vi "ExtractSeqWF.vi"(4 "yee delay":sgl, 5 "Correct Delay?":bool=TRUE, 6 "Acqiris delay":dbl, 7 "String":string, 8 "Offset":i32=11, 9 "Byte Swap":bool=TRUE) -> (1 "vert gain":sgl format="%.2e", 2 "Data Pts":i32, 3 "Data":i8[][](array[numeric]))   [LabVIEW 2022 SP3]
uses:
  -DigitizerRoutines/DigitizerGlobals.vi
panel:
  out "Hor offset":dbl format="%.2e"
  out "Trig Offset":dbl[](array[numeric]) format="%.2e"
  out "Trig Time":dbl[](array[numeric]) format="%.2e"
  out "#Data Bytes":i32
  out "Trig Time Array":i32
  out "Usr Text":i32
  out "Pts Per Screen":i32
  out "Nom Seg Count":i16
  out "WaveDesc":i32
  out "# of Segs":i32
  out "substring":string
  out "Nom bits":i32
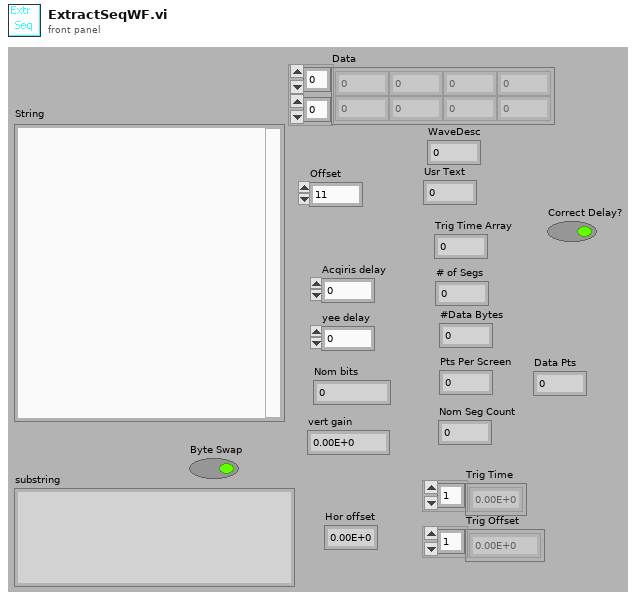
[diagram p1: front panel]
types:
  T1 = typedef "DigitizerSettings.ctl" = cluster{"Digitizer delay (us) ":dbl, "rf points per line":i32, "lines per plane":i32, "Samp Rate (Hz)":dbl, "Additional dig delay (us)":dbl, "Voltage Scale":dbl, "Pre-Looks":i32, "Offset delay (us)":dbl, "bits A/D":i8, "Avg Num":i32, "DigTimeOut":sgl, "Rel Dig Delay":sgl, "Dig Ch":i32, "LeCroyCluster":cluster{"LeCroy Channels":bool[], "LC read pt offset":dbl, "Sweep Avg":bool}, "Main Digitizer":T2, "Dig Config":T3, "Digitizer ID Cluster":T4, "Trigger Settings":cluster{"Trig Source":u16, "Trig Coupling":u16, "Trig Slope":u16, "Level (mV)":dbl}, "Bulk Acq":bool, "Bulk Start Indexes":i32[], "Data Ref RF":refnum<data-value>, "NI ID/Channel":cluster{"NI ID":refnum<k15>, "NI CH":i32}[], "Total Dig CH":i32, "Xtra Ann Trig delay (us)":dbl, "Fix Z Delay?":bool, "One Way Transmission?":bool, "Data Ref Log":refnum<data-value>}
  T2 = typedef "Digitizer.ctl" = enum16{"Acqiris Digitizer", "NI Digitizer", "LeCroy", "GaGe", "AlazarTech", "No Digitizer", "Teledyne"}
  T3 = typedef "DigConfig.ctl" = enum16{"Single channel", "2 Chans w/ 2 Acqiris", "2 Chans w/ 1 Acqiris", "5-CH Pulser New", "5-CH pulser w/ ann array", "5-pass style ann array", "Empty"}
  T4 = typedef "DigitizerID.ctl" = cluster{"Acqiris/Alazar/SP ID":u32[], "NI Instr Handles":refnum<k15>[], "LeCroy VISA":refnum<visa-resource-name>, "GaGe Handle":cluster{"Handle":u32, "Sample size":u32, "Resolution":i32, "Offset":i32, "Channels":u32, "Boards":u32}, "ATS Ref":string, "Acqiris Address":string[], "ADQRef":refnum<k24>, "adq_cu_ptr":refnum<k24>}
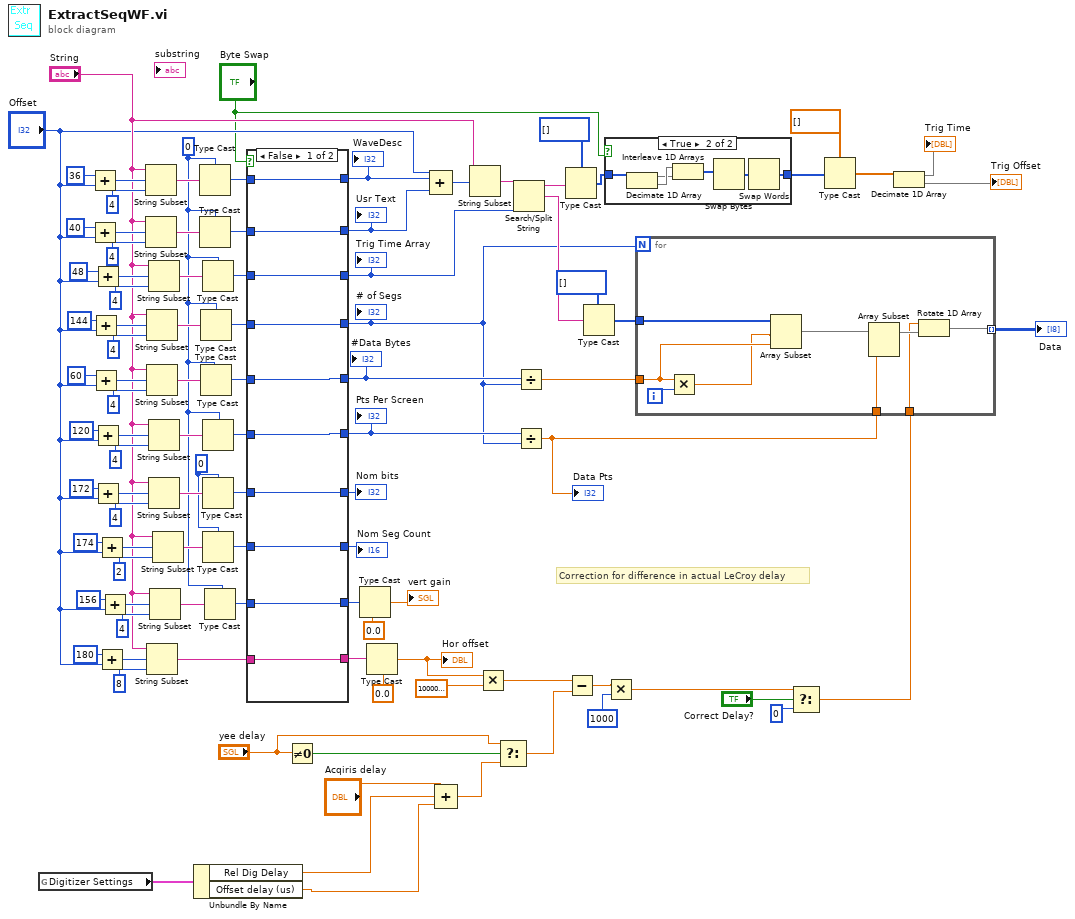
[diagram p0: block diagram]
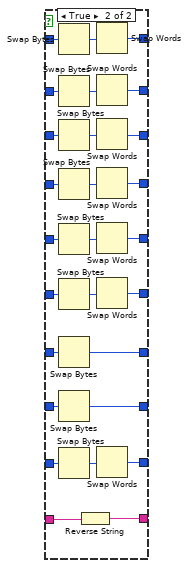
[diagram p3: hidden frame]
diagram:
  w17 = i16 0
  w27 = 0
  # "Correction for difference in actual LeCroy delay"
  n1 = global read "DigitizerGlobals.vi" "Digitizer Settings"() -> (w1:T1)
  n2 = Add(x=36, y="Offset") -> (x+y=w98:i32)
  n3 = Add(x=40, y="Offset") -> (x+y=w93:i32)
  n4 = Add(x=144, y="Offset") -> (x+y=w88:i32)
  n5 = Add(x=60, y="Offset") -> (x+y=w83:i32)
  n6 = Add(x=48, y="Offset") -> (x+y=w59:i32)
  n7 = Add(x=120, y="Offset") -> (x+y=w78:i32)
  n8 = Add(x=172, y="Offset") -> (x+y=w73:i32)
  n9 = Add(x=174, y="Offset") -> (x+y=w68:i32)
  n10 = Add(x=180, y="Offset") -> (x+y=w38:i32)
  n11 = Add(x=156, y="Offset") -> (x+y=w63:i32)
  n12 = String Subset(string="String", offset (0)=w98, length (rest)=4) -> (substring=w96:string)
  n13 = String Subset(string="String", offset (0)=w93, length (rest)=4) -> (substring=w91:string)
  n14 = String Subset(string="String", offset (0)=w88, length (rest)=4) -> (substring=w86:string)
  n15 = String Subset(string="String", offset (0)=w83, length (rest)=4) -> (substring=w81:string)
  n16 = String Subset(string="String", offset (0)=w38, length (rest)=8) -> (substring=w15:string)
  n17 = String Subset(string="String", offset (0)=w59, length (rest)=4) -> (substring=w57:string)
  n18 = String Subset(string="String", offset (0)=w78, length (rest)=4) -> (substring=w76:string)
  n19 = String Subset(string="String", offset (0)=w73, length (rest)=4) -> (substring=w71:string)
  n20 = String Subset(string="String", offset (0)=w63, length (rest)=4) -> (substring=w62:string)
  n21 = String Subset(string="String", offset (0)=w68, length (rest)=2) -> (substring=w66:string)
  n22 = Unbundle By Name(w1) -> ("Rel Dig Delay"=w2:sgl, "Offset delay (us)"=w3:dbl)
  n23 = Type Cast(type=w27, x=w96) -> (*(type *) &x=w97:i32)
  n24 = Type Cast(type=w27, x=w91) -> (*(type *) &x=w92:i32)
  n25 = Type Cast(type=w27, x=w86) -> (*(type *) &x=w87:i32)
  n26 = Type Cast(type=w27, x=w81) -> (*(type *) &x=w82:i32)
  n27 = Type Cast(type=w27, x=w57) -> (*(type *) &x=w58:i32)
  n28 = Type Cast(type=w27, x=w76) -> (*(type *) &x=w77:i32)
  n29 = Type Cast(type=w17, x=w71) -> (*(type *) &x=w72:i16)
  n30 = Type Cast(type=w17, x=w66) -> (*(type *) &x=w67:i16)
  n31 = Type Cast(type=w27, x=w62) -> (*(type *) &x=w44:i32)
  n32 = case shown="False" "Byte Swap" {
    tunnel: w97 -> [w110 w136]
    tunnel: w92 -> [w109 w134]
    tunnel: w87 -> [w107 w132]
    tunnel: w82 -> [w106 w130]
    tunnel: w77 -> [w105 w128]
    tunnel: w72 -> [w104 w127]
    tunnel: w67 -> [w103 w126]
    tunnel: w58 -> [w108 w123]
    tunnel: [w110 w122] -> w55
    tunnel: [w109 w121] -> w54
    tunnel: [w108 w120] -> w51
    tunnel: w44 -> [w102 w119]
    tunnel: [w102 w118] -> w43
    tunnel: [w106 w117] -> w33
    tunnel: [w105 w116] -> w32
    tunnel: [w107 w115] -> w31
    tunnel: [w103 w114] -> w29
    tunnel: [w104 w113] -> w26
    tunnel: w15 -> [w101 w112]
    tunnel: [w101 w111] -> w14
    frame False {
    }
    frame True {
      n33 = Swap Bytes(anything=w136) -> (byte swapped=w137:i32)
      n34 = Swap Bytes(anything=w134) -> (byte swapped=w135:i32)
      n35 = Swap Bytes(anything=w123) -> (byte swapped=w124:i32)
      n36 = Swap Bytes(anything=w132) -> (byte swapped=w133:i32)
      n37 = Swap Bytes(anything=w130) -> (byte swapped=w131:i32)
      n38 = Swap Bytes(anything=w128) -> (byte swapped=w129:i32)
      n39 = Swap Bytes(anything=w127) -> (byte swapped=w113:i16)
      n40 = Swap Bytes(anything=w126) -> (byte swapped=w114:i16)
      n41 = Swap Bytes(anything=w119) -> (byte swapped=w125:i32)
      n42 = Reverse String(1:w112) -> (0:w111:string)
      n43 = Swap Words(1:w137) -> (0:w122:i32)
      n44 = Swap Words(1:w135) -> (0:w121:i32)
      n45 = Swap Words(1:w124) -> (0:w120:i32)
      n46 = Swap Words(1:w133) -> (0:w115:i32)
      n47 = Swap Words(1:w131) -> (0:w117:i32)
      n48 = Swap Words(1:w129) -> (0:w116:i32)
      n49 = Swap Words(1:w125) -> (0:w118:i32)
    }
  }
  "Nom bits" <- w26
  "# of Segs" <- w31
  "WaveDesc" <- w55
  "Nom Seg Count" <- w29
  "Pts Per Screen" <- w32
  "Usr Text" <- w54
  "Trig Time Array" <- w51
  "#Data Bytes" <- w33
  n50 = Not Equal To 0?(x="yee delay") -> (x != 0?=w11:bool)
  n51 = Type Cast(type=sgl 0.0, x=w43) -> (*(type *) &x=→"vert gain":sgl)
  n52 = Type Cast(type=0.0, x=w14) -> (*(type *) &x=w23:dbl)
  "Hor offset" <- w23
  n53 = Compound Arithmetic op=ADD("Offset", w55, w54) -> (w53:i32)
  n54 = Compound Arithmetic op=ADD("Acqiris delay", w2, w3) -> (w10:dbl)
  n55 = String Subset(string="String", offset (0)=w53) -> (substring=w52:string)  [unwired: 1 out]
  n56 = Multiply(x=w23, y=1000000.0) -> (x*y=w19:dbl)
  n57 = Select(t="yee delay", s=w11, f=w10) -> (s? t:f=w9:dbl)
  n58 = Search/Split String(string=w52, offset (0)=w51) -> (substring before match=w49:string, match + rest of string=w50:string)  [unwired: 2 out]
  n59 = Divide(x=w33, y=w31) -> (x/y=w41:dbl)
  n60 = Divide(x=w32, y=w31) -> (x/y=w30:dbl)
  "Data Pts" <- w30
  n61 = Type Cast(type=i32[] [], x=w49) -> (*(type *) &x=w13:i32[])
  n62 = Subtract(x=w19, y=w9) -> (x-y=w21:dbl)
  n63 = Type Cast(type=i8[] [], x=w50) -> (*(type *) &x=w34:i8[])
  n64 = case shown="True" "Byte Swap" {
    tunnel: w13 -> [w138 w141]
    tunnel: [w138 w139] -> w45
    frame False {
    }
    frame True {
      n65 = Decimate 1D Array(w141) -> (w142:i32[], w143:i32[])
      n66 = Interleave 1D Arrays(w143, w142) -> (w140:i32[])
      n67 = Swap Bytes(anything=w140) -> (byte swapped=w144:i32[])
      n68 = Swap Words(1:w144) -> (0:w139:i32[])
    }
  }
  n69 = Multiply(x=w21, y=1000) -> (x*y=w4:dbl)
  n70 = Select(t=w4, s="Correct Delay?", f=0) -> (s? t:f=w7:dbl)
  n71 = for {
    N: w31 -> [_]
    tunnel: w41 -> [w151]
    tunnel: w34 -> [w152]
    tunnel: [w146] -> w24 mode=indexing
    tunnel: w30 -> [w148]
    tunnel: w7 -> [w145]
    i -> [w153]
    n72 = Multiply(x=w151, y=w153) -> (x*y=w150:dbl)
    n73 = Array Subset(array=w152, index=w150, length=w151) -> (w149:i8[])
    n74 = Array Subset(array=w149, length=w148) -> (w147:i8[])  [unwired: 1 in]
    n75 = Rotate 1D Array(1:w147, 2:w145) -> (0:w146:i8[])
  }
  "Data" <- w24
  n76 = Type Cast(type=dbl[] [], x=w45) -> (*(type *) &x=w35:dbl[])
  n77 = Decimate 1D Array(w35) -> (→"Trig Time":dbl[], →"Trig Offset":dbl[])
